vi "RGB to XYZ.vi"(9 "Blue":i16, 10 "Green":i16, 11 "Red":i16) -> (1 "Z":dbl, 2 "Y":dbl, 3 "X":dbl)   [LabVIEW 2016, in "AMS TS3472 Light Sensor.lvlib" / "AMS TCS3472.lvclass"]
uses:
  AMS TCS3472.lvclass
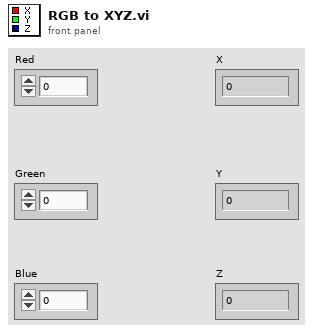
[diagram p1: front panel]
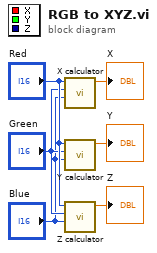
[diagram p0: block diagram]
diagram:
  n1 = call "X calculator.vi"("Blue"="Blue", "Green"="Green", "Red"="Red") -> ("X"=→"X":dbl)  [unwired: 8 in]
  n2 = call "Y calculator.vi"("Blue"="Blue", "Green"="Green", "Red"="Red") -> ("Y"=→"Y":dbl)  [unwired: 8 in]
  n3 = call "Z calculator.vi"("Blue"="Blue", "Green"="Green", "Red"="Red") -> ("Z"=→"Z":dbl)  [unwired: 8 in]
